vi "Enum Convert Into String.vi"() -> ()   [LabVIEW 2020]
panel:
  out "resulting string":string
  in  "Enum":enum16{"Pardeep", "Pooja", "Mandeep"}(ring)
  # "Enum Convert Into String"
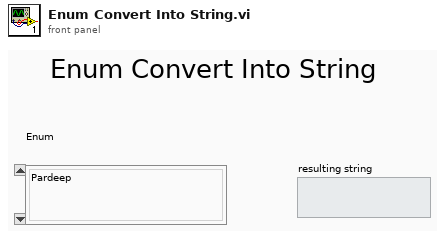
[diagram p1: front panel]
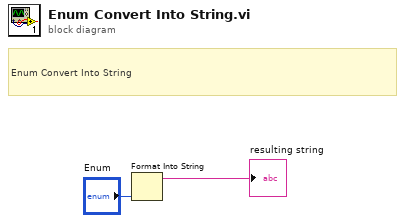
[diagram p0: block diagram]
diagram:
  # "Enum Convert Into String"
  n1 = Format Into String "Format Into String"("Enum") -> (resulting string=→"resulting string":string)  [unwired: 3 in, 1 out]
